vi "loadGraph.vi"(1 "filePath":path, 2 "graphics":refnum<class "Graphics.lvclass">, 3 "grid":refnum<class "Grid.lvclass">, 5 "error in (no error)":errorcluster) -> (14 "reference out":refnum<class "Graph.lvclass">, 15 "succeeded":bool, 16 "String":string, 17 "NodesBounds":T1 {"height" format="%.2f"; "width" format="%.2f"; "y" format="%.2f"; "x" format="%.2f"}, 19 "error out":errorcluster)   [LabVIEW 2014, in "Graph.lvclass"]
doc: "Save to File"
uses:
  <resource>/Framework/Providers/Open_GDS/UML/Graph_class/Graph.lvclass
  <resource>/Framework/Providers/Open_GDS/UML/General/Rectangle/Rectangle Rectangle2D.ctl
  <resource>/Framework/Providers/Open_GDS/UML/Grid_class/Grid.lvclass
  <resource>/Framework/Providers/Open_GDS/UML/Graphics_class/Graphics.lvclass
  <resource>/Framework/Providers/Open_GDS/UML/AbstractNode_class/AbstractNode.lvclass
  <resource>/Framework/Providers/Open_GDS/UML/AbstractEdge_class/AbstractEdge.lvclass
  <resource>/Framework/Providers/Open_GDS/UML/Graph_class/FileContent.ctl
  <resource>/Framework/Providers/Open_GDS/UML/PointNode_class/PointNode.lvclass
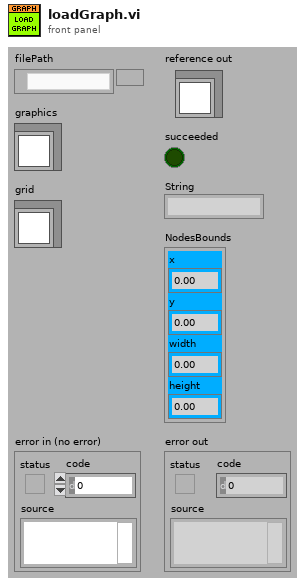
[diagram p1: front panel]
types:
  T1 = typedef "Rectangle Rectangle2D.ctl" = cluster{"x":dbl, "y":dbl, "width":dbl, "height":dbl}
  T2 = cluster{"graph":refnum<class "Graph.lvclass">, "succeeded":bool, "nodeInfo":cluster{"NodeType":string[], "ParentIndex":i32[], "ChildernIndexies":cluster{i32[]}[], "FlattenData":string[]}, "edgeInfo":cluster{"EdgeType":string[], "StartNodeIndex":i32[], "EndNodeIndex":i32[], "FlattenData":string[]}, "nodes":refnum<class "AbstractNode.lvclass">[], "edges":refnum<class "AbstractEdge.lvclass">[], "DiagramData":string, "bounds":T1, "diagramType":string}
  T3 = typedef "Graph.lvclass/FileContent.ctl" = cluster{"Version":string, "DiagramType":string, "DiagramData":string, "Nodes":cluster{"NodeType":string[], "ParentIndex":i32[], "ChildernIndexies":cluster{i32[]}[], "FlattenData":string[]}, "Edges":cluster{"EdgeType":string[], "StartNodeIndex":i32[], "EndNodeIndex":i32[], "FlattenData":string[]}}
  T4 = enum16{"read/write", "read-only", "write-only", "write-only (truncate)"}
  T5 = enum16{"None", "Class", "Sequency", "State", "UseCase"}
  T6 = cluster{"NodeType":string[], "ParentIndex":i32[], "ChildernIndexies":cluster{i32[]}[], "FlattenData":string[]}
  T7 = cluster{"EdgeType":string[], "StartNodeIndex":i32[], "EndNodeIndex":i32[], "FlattenData":string[]}
  T8 = cluster{"TYPEDEF-FileSaveVersion":enum16{"A"}, "diagramType":enum16{"None", "Class", "Sequency", "State", "UseCase"}, string, "nodeInfo":cluster{"NodeType":string[], "ParentIndex":i32[], "ChildernIndexies":cluster{i32[]}[], "FlattenData":string[]}, "edgeInfo":cluster{"EdgeType":string[], "StartNodeIndex":i32[], "EndNodeIndex":i32[], "FlattenData":string[]}}
  T9 = cluster{"diagramType":enum16{"None", "Class", "Sequency", "State", "UseCase"}, "nodeInfo":cluster{"NodeType":string[], "ParentIndex":i32[], "ChildernIndexies":cluster{i32[]}[], "FlattenData":string[]}, "edgeInfo":cluster{"EdgeType":string[], "StartNodeIndex":i32[], "EndNodeIndex":i32[], "FlattenData":string[]}}
  T10 = typedef "Graph.lvclass/ClassAttributes.ctl" = cluster{"NODE_PROT":refnum<class "AbstractNode.lvclass">[], "NodeNames":string[], "EDGE_PROT":refnum<class "AbstractEdge.lvclass">[], "EdgeNames":string[], "GraphTypes":refnum<class "Graph.lvclass">[], "GraphTypeNames":string[], "NodeTypes":refnum<class "AbstractNode.lvclass">[], "EdgeTypes":refnum<class "AbstractEdge.lvclass">[]}
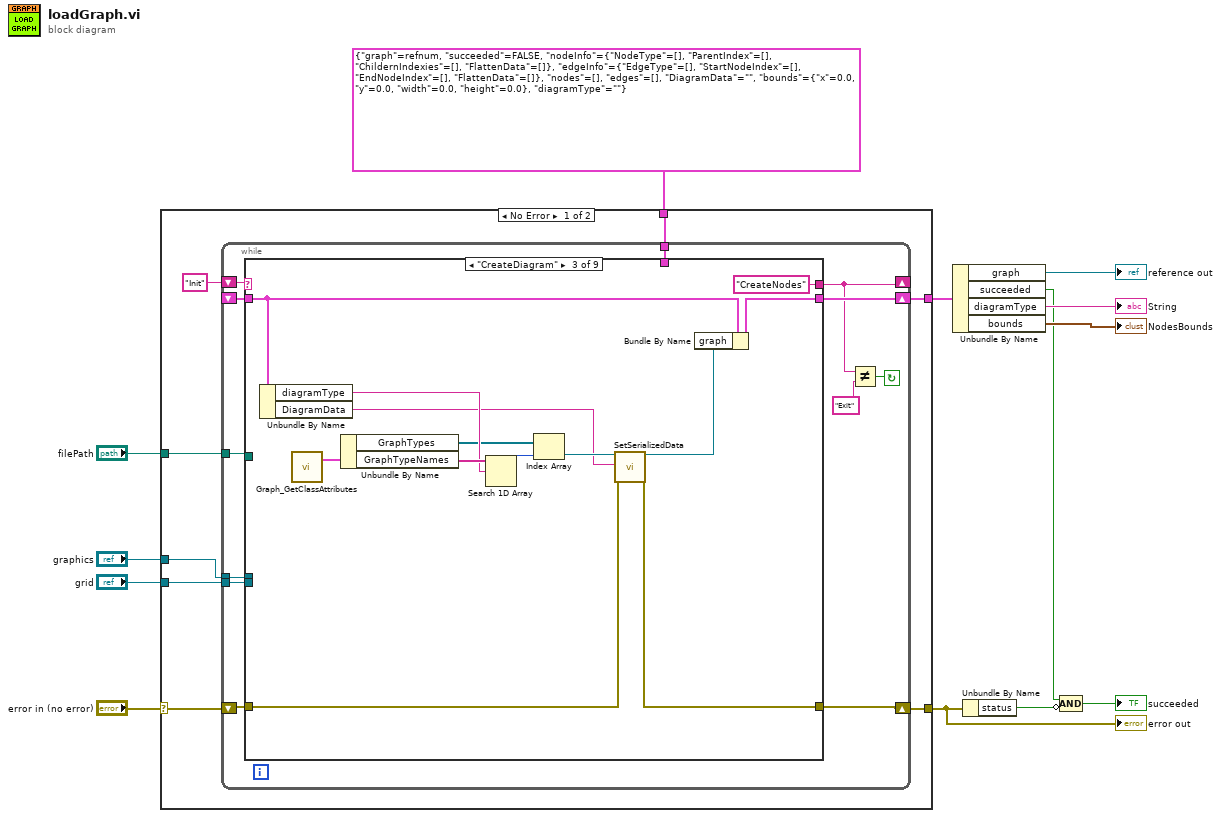
[diagram p0: block diagram]
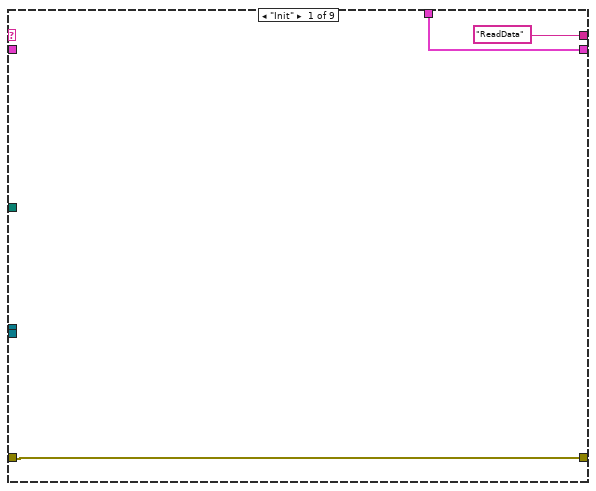
[diagram p2: hidden frame]
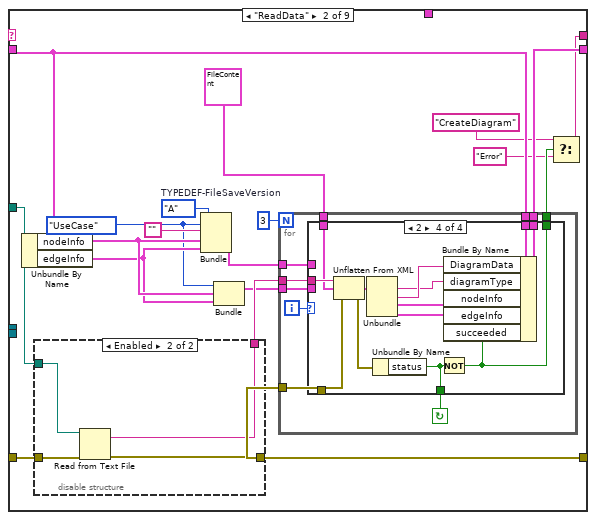
[diagram p3: hidden frame]
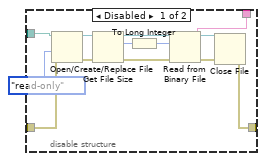
[diagram p4: hidden frame]
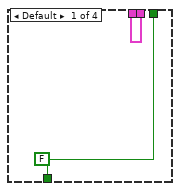
[diagram p5: hidden frame]
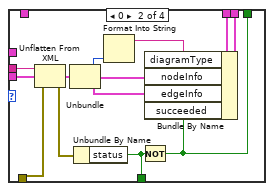
[diagram p6: hidden frame]
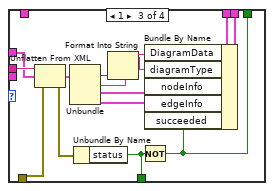
[diagram p7: hidden frame]
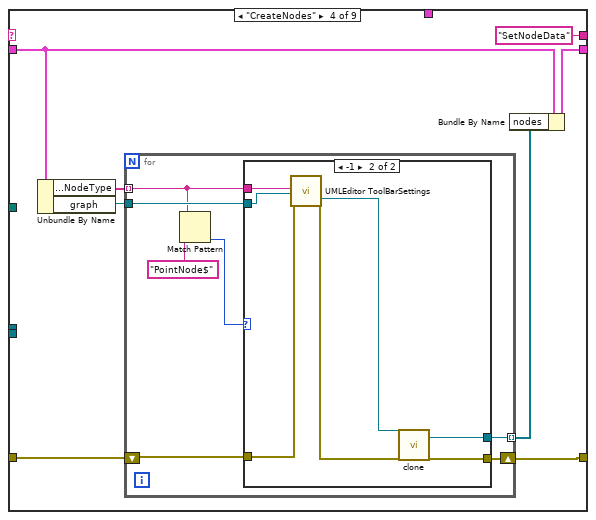
[diagram p8: hidden frame]
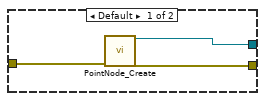
[diagram p9: hidden frame]
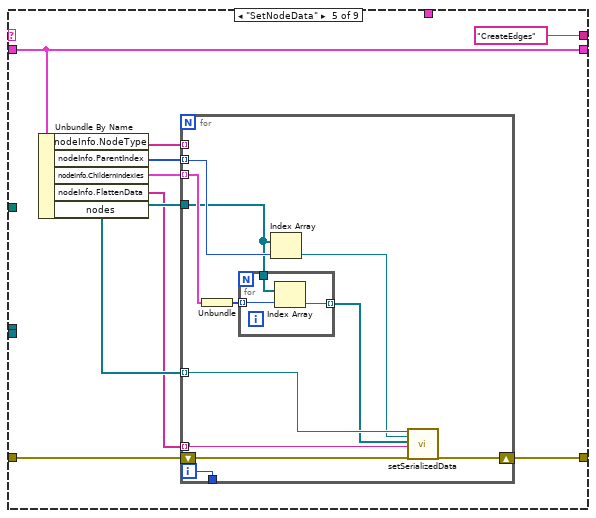
[diagram p10: hidden frame]
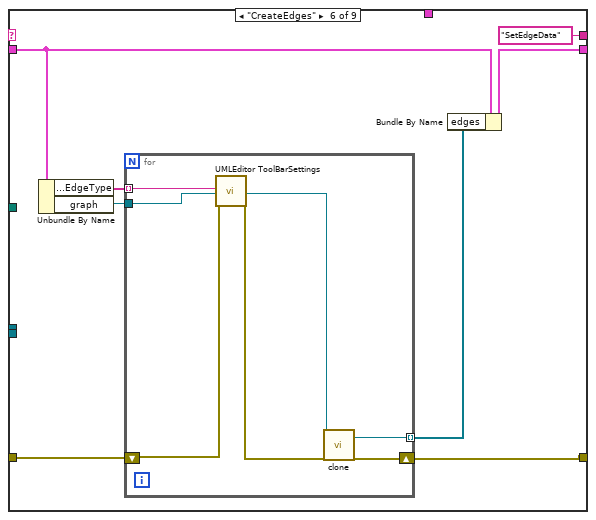
[diagram p11: hidden frame]
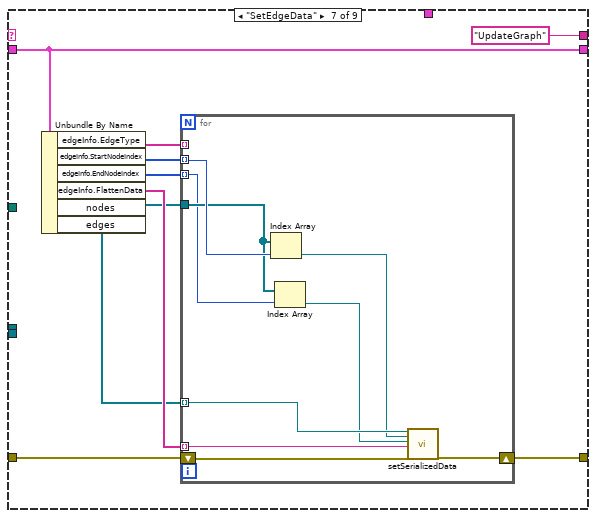
[diagram p12: hidden frame]
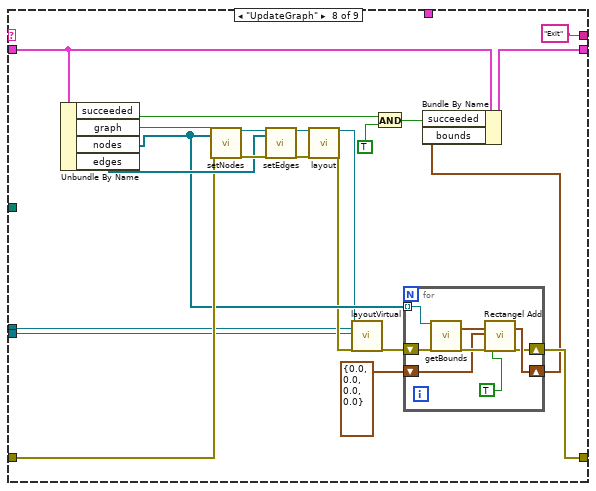
[diagram p13: hidden frame]
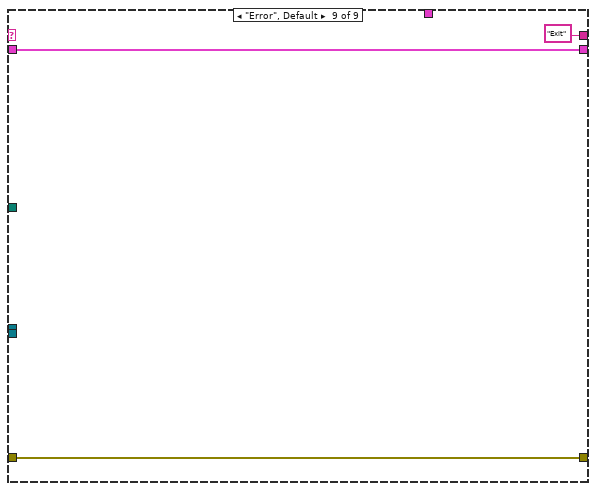
[diagram p14: hidden frame]
diagram:
  n1 = case shown="No Error" "error in (no error)" {
    selector: "error in (no error)" -> [w18 w253]
    tunnel: [w17 w253] -> w5
    tunnel: "filePath" -> [w21 _]
    tunnel: [w19 _] -> w11
    tunnel: "graphics" -> [w16 _]
    tunnel: "grid" -> [w15 _]
    tunnel: T2 {"graph"=refnum, "succeeded"=FALSE, "nodeInfo"={"NodeType"=[], "ParentIndex"=[], "ChildernIndexies"=[], "FlattenData"=[]}, "edgeInfo"={"EdgeType"=[], "StartNodeIndex"=[], "EndNodeIndex"=[], "FlattenData"=[]}, "nodes"=[], "edges"=[], "DiagramData"="", "bounds"={"x"=0.0, "y"=0.0, "width"=0.0, "height"=0.0}, "diagramType"=""} ("localData") -> [w14 _]
    frame No Error {
      n2 = while {
        tunnel: w21 -> [w33]
        shift-right: [w28] -> _
        shift-left: "Init" -> [w32]
        shift-right: [w31] -> w19
        shift-left: _ -> [w27]
        shift-right: [w25] -> w17
        shift-left: w18 -> [w26]
        tunnel: w16 -> [w24]
        tunnel: w15 -> [w23]
        tunnel: w14 -> [w22]
        stop <- w29 continue-if-true
        n3 = case shown="\"CreateDiagram\"" w32 {
          tunnel: w26 -> [w36 w48 w127 w143 w164 w191 w204 w235 w252]
          tunnel: w33 -> [_ w47 _ _ _ _ _ _ _]
          tunnel: [w36 w54 w126 w138 w163 w188 w203 w227 w252] -> w25
          tunnel: [w34 w52 w135 w141 w171 w190 w210 w233 w250] -> w31
          tunnel: ["ReadData" w49 "CreateNodes" "SetNodeData" "CreateEdges" ("y") "SetEdgeData" "UpdateGraph" ("y") "Exit" ("y") "Exit" ("y")] -> w28
          tunnel: w27 -> [_ w51 w136 w140 w171 w189 w210 w232 w250]
          tunnel: w24 -> [_ _ _ _ _ _ _ w221 _]
          tunnel: w23 -> [_ _ _ _ _ _ _ w220 _]
          tunnel: w22 -> [w34 _ _ _ _ _ _ _ _]
          frame "Init" {
          }
          frame "ReadData" {
            w43 = enum16{"A"}."A"  # TYPEDEF-FileSaveVersion
            w38 = T5."UseCase" ("diagramType")
            n4 = Unbundle By Name(w51) -> ("nodeInfo"=w41:T6, "edgeInfo"=w40:T7)
            n5 = disable-structure shown="Enabled" {
              disable-tunnel: [w60 w69] -> w55
              disable-tunnel: [w59 w70] -> w54
              disable-tunnel: w48 -> [w58 w72]
              disable-tunnel: w47 -> [w57 w71]
              frame Disabled {
                n6 = Open/Create/Replace File(file path (use dialog)=w57, error in=w58, access (0:read/write)=T4."read-only" ("open mode (0)")) -> (refnum out=w63:refnum<file>, error out=w64:errorcluster)  [unwired: 3 in, 1 out]
                n7 = Get File Size(file=w63, error in=w64) -> (refnum out=w65:refnum<file>, size (in bytes)=w56:i64, 0:w66:errorcluster)
                n8 = To Long Integer(number=w56) -> (32bit integer=w62:i32)
                n9 = Read from Binary File(8:w66, 10:w62, 11:w65) -> (0:w68:errorcluster, 2:w60:string, 3:w67:refnum<file>)  [unwired: 4 out]
                n10 = Close File(refnum=w67, error in=w68) -> (error out=w59:errorcluster)  [unwired: 1 out]
              }
              frame Enabled {
                n11 = Read from Text File(file (use dialog)=w71, error in=w72) -> (text=w69:string, error out=w70:errorcluster)  [unwired: 2 in, 2 out]
              }
            }
            n12 = Bundle("TYPEDEF-FileSaveVersion"=w43, "diagramType"=w38, "", "nodeInfo"=w41, "edgeInfo"=w40) -> (w42:T8)  [unwired: 1 out]
            n13 = Bundle("diagramType"=w38, "nodeInfo"=w41, "edgeInfo"=w40) -> (w53:T9)  [unwired: 1 out]
            n14 = for {
              N: 3 -> [_]
              tunnel: w55 -> [w82]
              tunnel: w54 -> [w81]
              tunnel: w53 -> [w80]
              tunnel: [w79] -> w52
              tunnel: w51 -> [w78]
              tunnel: [w77] -> w50
              tunnel: w42 -> [w75]
              tunnel: T3 {"Version"="", "DiagramType"="", "DiagramData"="", "Nodes"={"NodeType"=[], "ParentIndex"=[], "ChildernIndexies"=[], "FlattenData"=[]}, "Edges"={"EdgeType"=[], "StartNodeIndex"=[], "EndNodeIndex"=[], "FlattenData"=[]}} ("cluster") -> [w73]
              i -> [w76]
              stop <- w74 continue-if-true
              n15 = case shown="2" w76 {
                tunnel: w82 -> [_ w97 w111 w124]
                tunnel: w81 -> [_ w96 w110 w123]
                tunnel: w80 -> [_ w94 _ _]
                tunnel: [w84 w91 w108 w121] -> w79
                tunnel: w78 -> [w84 w90 w107 w120]
                tunnel: [w83 w87 w104 w117] -> w77
                tunnel: [w83 w88 w105 w118] -> w74
                tunnel: w75 -> [_ _ w103 _]
                tunnel: w73 -> [_ _ _ w113]
                frame Default {
                  w83 = FALSE ("status")
                }
                frame 0 {
                  n16 = Unflatten From XML(xml string=w97, type=w94, error in (no error)=w96) -> (value=w95:T9, error out=w89:errorcluster)
                  n17 = Unbundle(w95) -> ("diagramType"=w86:T5, "nodeInfo"=w93:T6, "edgeInfo"=w92:T7)
                  n18 = Unbundle By Name(w89) -> ("status"=w88:bool)
                  n19 = Format Into String(w86) -> (resulting string=w85:string)  [unwired: 3 in, 1 out]
                  n20 = Not(x=w88) -> (.not. x?=w87:bool)
                  n21 = Bundle By Name(cluster=w90, "diagramType"=w85, "nodeInfo"=w93, "edgeInfo"=w92, "succeeded"=w87) -> (w91:T2)
                }
                frame 1 {
                  n22 = Unflatten From XML(xml string=w111, type=w103, error in (no error)=w110) -> (value=w109:T8, error out=w106:errorcluster)
                  n23 = Unbundle(w109) -> ("diagramType"=w99:T5, w100:string, "nodeInfo"=w102:T6, "edgeInfo"=w101:T7)  [unwired: 1 out]
                  n24 = Unbundle By Name(w106) -> ("status"=w105:bool)
                  n25 = Format Into String(w99) -> (resulting string=w98:string)  [unwired: 3 in, 1 out]
                  n26 = Not(x=w105) -> (.not. x?=w104:bool)
                  n27 = Bundle By Name(cluster=w107, "DiagramData"=w100, "diagramType"=w98, "nodeInfo"=w102, "edgeInfo"=w101, "succeeded"=w104) -> (w108:T2)
                }
                frame 2 {
                  n28 = Unflatten From XML(xml string=w124, type=w113, error in (no error)=w123) -> (value=w122:T3, error out=w119:errorcluster)
                  n29 = Unbundle(w122) -> ("DiagramType"=w112:string, "DiagramData"=w114:string, "Nodes"=w116:T6, "Edges"=w115:T7)  [unwired: 1 out]
                  n30 = Unbundle By Name(w119) -> ("status"=w118:bool)
                  n31 = Not(x=w118) -> (.not. x?=w117:bool)
                  n32 = Bundle By Name(cluster=w120, "DiagramData"=w114, "diagramType"=w112, "nodeInfo"=w116, "edgeInfo"=w115, "succeeded"=w117) -> (w121:T2)
                }
              }
            }
            n33 = Select(t="CreateDiagram" ("y"), s=w50, f="Error" ("y")) -> (s? t:f=w49:string)
          }
          frame "CreateDiagram" {
            n34 = Unbundle By Name(w136) -> ("diagramType"=w132:string, "DiagramData"=w128:string)
            n35 = call <resource>:"Graph_GetClassAttributes.vi"() -> ("Class attribute"=w134:T10)  [unwired: 16 in, 3 out]
            n36 = Unbundle By Name(w134) -> ("GraphTypes"=w131:refnum<class "Graph.lvclass">[], "GraphTypeNames"=w133:string[])
            n37 = Search 1D Array(1D array=w133, element=w132) -> (index of element=w130:i32)  [unwired: 1 in]
            n38 = Index Array(array=w131, index=w130) -> (element=w129:refnum<class "Graph.lvclass">)
            n39 = call-dynamic "SetSerializedData.vi"("reference in"=w129, "SerializedData(XML)"=w128, "error in (no error)"=w127) -> ("reference out"=w125:refnum<class "Graph.lvclass">, "error out"=w126:errorcluster)  [unwired: 15 in]
            n40 = Bundle By Name(cluster=w136, "graph"=w125) -> (w135:T2)
          }
          frame "CreateNodes" {
            n41 = Unbundle By Name(w140) -> ("nodeInfo.NodeType"=w144:string[], "graph"=w139:refnum<class "Graph.lvclass">)
            n42 = for {
              tunnel: w144 -> [w146] mode=indexing
              shift-right: [w149] -> w138
              shift-left: w143 -> [w151]
              tunnel: [w152] -> w142 mode=indexing
              tunnel: w139 -> [w150]
              n43 = Match Pattern(string=w146, regular expression="PointNode$") -> (offset past match=w147:i32)  [unwired: 4 out]
              n44 = case shown="-1" w147 {
                tunnel: [w154 w162] -> w152
                tunnel: w146 -> [_ w161]
                tunnel: w151 -> [w155 w160]
                tunnel: w150 -> [_ w158]
                tunnel: [w153 w156] -> w149
                frame Default {
                  n45 = call <resource>:"PointNode_Create.vi"("error in (no error)"=w155) -> ("reference out"=w154:refnum<class "PointNode.lvclass">, "error out"=w153:errorcluster)  [unwired: 1 in, 16 out]
                }
                frame -1 {
                  n46 = call <resource>:"UMLEditor ToolBarSettings.vi"("NodeName/EdgeName(empty=not in use)"=w161, "graph(only used with className input)"=w158, "error in (no error)"=w160) -> ("prototypeNode"=w157:refnum<class "AbstractNode.lvclass">, "error out"=w159:errorcluster)  [unwired: 1 in, 14 out]
                  n47 = call-dynamic "clone.vi"("reference"=w157, "error in (no error)"=w159) -> ("clonedAbstractNode"=w162:refnum<class "AbstractNode.lvclass">, "error out"=w156:errorcluster)  [unwired: 15 in, 1 out]
                }
              }
            }
            n48 = Bundle By Name(cluster=w140, "nodes"=w142) -> (w141:T2)
          }
          frame "SetNodeData" {
            n49 = Unbundle By Name(w171) -> ("nodeInfo.NodeType"=w169:string[], "nodeInfo.ParentIndex"=w168:i32[], "nodeInfo.ChildernIndexies"=w167:cluster{i32[]}[], "nodeInfo.FlattenData"=w165:string[], "nodes"=w166:refnum<class "AbstractNode.lvclass">[])
            n50 = for {
              tunnel: w169 -> [_] mode=indexing
              tunnel: w168 -> [w182] mode=indexing
              tunnel: w167 -> [w181] mode=indexing
              tunnel: w166 -> [w180]
              tunnel: w166 -> [w178] mode=indexing
              tunnel: w165 -> [w174] mode=indexing
              shift-right: [w175] -> w163
              shift-left: w164 -> [w173]
              tunnel: [w172] -> _
              i -> [w172]
              n51 = Unbundle(w181) -> (w179:i32[])
              n52 = for {
                tunnel: w180 -> [w185]
                tunnel: w179 -> [w184] mode=indexing
                tunnel: [w183] -> w176 mode=indexing
                n53 = Index Array(array=w185, index=w184) -> (element=w183:refnum<class "AbstractNode.lvclass">)
              }
              n54 = Index Array(array=w180, index=w182) -> (element=w177:refnum<class "AbstractNode.lvclass">)
              n55 = call-dynamic "setSerializedData.vi"("reference"=w178, "parent"=w177, "children"=w176, "xmlOut"=w174, "error in (no error)"=w173) -> ("error out"=w175:errorcluster)  [unwired: 13 in, 1 out]
            }
          }
          frame "CreateEdges" {
            n56 = Unbundle By Name(w189) -> ("edgeInfo.EdgeType"=w192:string[], "graph"=w187:refnum<class "Graph.lvclass">)
            n57 = for {
              tunnel: w192 -> [w199] mode=indexing
              shift-right: [w200] -> w188
              shift-left: w191 -> [w198]
              tunnel: w187 -> [w196]
              tunnel: [w194] -> w186 mode=indexing
              n58 = call <resource>:"UMLEditor ToolBarSettings.vi"("NodeName/EdgeName(empty=not in use)"=w199, "graph(only used with className input)"=w196, "error in (no error)"=w198) -> ("prototypeEdge"=w195:refnum<class "AbstractEdge.lvclass">, "error out"=w197:errorcluster)  [unwired: 1 in, 14 out]
              n59 = call-dynamic "clone.vi"("reference"=w195, "error in (no error)"=w197) -> ("clonedEdge"=w194:refnum<class "AbstractEdge.lvclass">, "error out"=w200:errorcluster)  [unwired: 15 in, 1 out]
            }
            n60 = Bundle By Name(cluster=w189, "edges"=w186) -> (w190:T2)
          }
          frame "SetEdgeData" {
            n61 = Unbundle By Name(w210) -> ("edgeInfo.EdgeType"=w208:string[], "edgeInfo.StartNodeIndex"=w207:i32[], "edgeInfo.EndNodeIndex"=w206:i32[], "edgeInfo.FlattenData"=w205:string[], "nodes"=w202:refnum<class "AbstractNode.lvclass">[], "edges"=w201:refnum<class "AbstractEdge.lvclass">[])
            n62 = for {
              tunnel: w208 -> [_] mode=indexing
              tunnel: w207 -> [w219] mode=indexing
              tunnel: w206 -> [w213] mode=indexing
              tunnel: w202 -> [w218]
              tunnel: w201 -> [w217] mode=indexing
              tunnel: w205 -> [w212] mode=indexing
              shift-right: [w214] -> w203
              shift-left: w204 -> [w211]
              n63 = Index Array(array=w218, index=w219) -> (element=w216:refnum<class "AbstractNode.lvclass">)
              n64 = Index Array(array=w218, index=w213) -> (element=w215:refnum<class "AbstractNode.lvclass">)
              n65 = call-dynamic "setSerializedData.vi"("reference"=w217, "startNode"=w216, "endNode"=w215, "xmlOut"=w212, "error in (no error)"=w211) -> ("error out"=w214:errorcluster)  [unwired: 13 in, 1 out]
            }
          }
          frame "UpdateGraph" {
            n66 = Unbundle By Name(w232) -> ("succeeded"=w231:bool, "graph"=w241:refnum<class "Graph.lvclass">, "nodes"=w226:refnum<class "AbstractNode.lvclass">[], "edges"=w238:refnum<class "AbstractEdge.lvclass">[])
            n67 = call-dynamic "setNodes.vi"("reference"=w241, "nodes"=w226, "error in (no error)"=w235) -> ("reference out"=w240:refnum<class "Graph.lvclass">, "error out"=w239:errorcluster)  [unwired: 15 in]
            n68 = call-dynamic "setEdges.vi"("reference"=w240, "edges"=w238, "error in (no error)"=w239) -> ("reference out"=w237:refnum<class "Graph.lvclass">, "error out"=w236:errorcluster)  [unwired: 15 in]
            n69 = call-dynamic "layout.vi"("reference"=w237, "error in (no error)"=w236) -> ("reference out"=w223:refnum<class "Graph.lvclass">, "error out"=w222:errorcluster)  [unwired: 16 in]
            n70 = call <resource>:"layoutVirtual.vi"("reference"=w223, "graphics"=w221, "grid"=w220, "error in (no error)"=w222) -> ("error out"=w224:errorcluster)  [unwired: 15 out]
            n71 = And(x=w231, y=TRUE) -> (x .and. y?=w230:bool)
            n72 = for {
              shift-right: [w244] -> w227
              shift-left: w224 -> [w243]
              shift-right: [w245] -> w225
              shift-left: T1 {"x"=0.0, "y"=0.0, "width"=0.0, "height"=0.0} ("boundsAdded") -> [w246]
              tunnel: w226 -> [w242] mode=indexing
              n73 = call-dynamic "getBounds.vi"("reference"=w242, "error in (no error)"=w243) -> ("bounds"=w249:T1, "error out"=w248:errorcluster)  [unwired: 15 in, 1 out]
              n74 = call <resource>:"Rectangel Add.vi"("bounds1"=w249, "bounds2"=w246, "error in (no error)"=w248, "useAbsoluteCordinates(False)"=TRUE) -> ("boundsAdded"=w245:T1, "error out"=w244:errorcluster)  [unwired: 1 in, 13 out]
            }
            n75 = Bundle By Name(cluster=w232, "succeeded"=w230, "bounds"=w225) -> (w233:T2)
          }
          frame "Error", Default {
          }
        }
        n76 = Not Equal?(x=w28, y="Exit") -> (x != y?=w29:bool)
      }
    }
    frame Error {
    }
  }
  "error out" <- w5
  n77 = Unbundle By Name(w11) -> ("graph"=→"reference out":refnum<class "Graph.lvclass">, "succeeded"=w3:bool, "diagramType"=→"String":string, "bounds"=→"NodesBounds":T1)
  n78 = Unbundle By Name(w5) -> ("status"=w4:bool)
  n79 = Compound Arithmetic op=AND(w3, invert w4) -> (→"succeeded":bool)
